vi "MyGlobal-Global.vi"() -> ()   [LabVIEW 2017]
panel:
  in  "布尔":bool
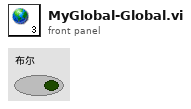
[diagram p1: front panel]
diagram:
